vi "Shutdown.vi"(8 "error in (no error)":errorcluster, 9 "Message Data":variant, 10 "Name":string, 11 "Controller in":refnum<class "Controller.lvclass">) -> (0 "error out":errorcluster, 3 "Controller out":refnum<class "Controller.lvclass">)   [LabVIEW 2020, in "Controller.lvlib" / "Controller.lvclass"]
uses:
  Controller.lvclass
  RPC/TypeDefs/Request.ctl
  Controller.lvclass/Controller.ctl
  RPC.lvlib
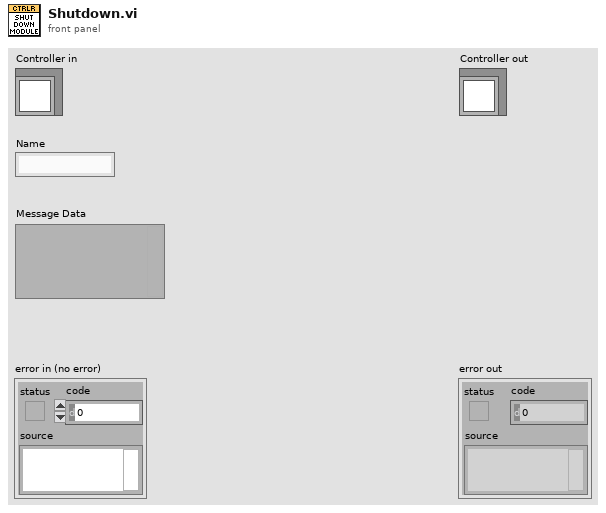
[diagram p1: front panel]
types:
  T1 = typedef "RPC.lvlib/Request.ctl" = cluster{"Method":string, "Params":variant}
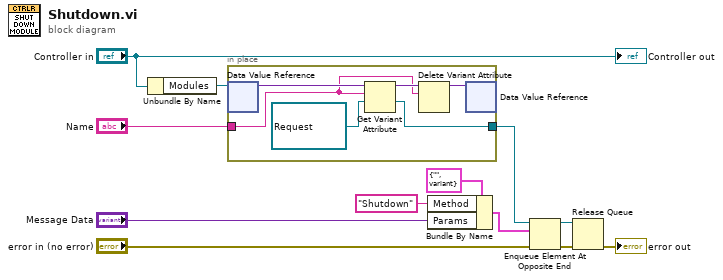
[diagram p0: block diagram]
diagram:
  n1 = Unbundle By Name("Controller in") -> ("Modules"=w10:refnum<data-value>)
  n2 = in-place {
    in-place-border: "Name" -> [w14]
    in-place-border: [w15] -> w2
    n3 = in-place-dvr #1(w10) -> (w17:variant)  [unwired: 1 out]
    n4 = Get Variant Attribute(Variant=w17, name=w14, default value (empty Variant)=refnum<queue> refnum ("queue out")) -> (duplicate Variant=w16:variant, value=w15:refnum<queue>)  [unwired: 1 in, 2 out]
    n5 = Delete Variant Attribute(6:w14, 7:w16) -> (3:w18:variant)  [unwired: 1 in, 2 out]
    n6 = in-place-dvr #1(w18) -> ()  [unwired: 2 out]
  }
  n7 = Bundle By Name(cluster=T1 {"Method"="", "Params"=variant} ("element"), "Method"="Shutdown" ("Message"), "Params"="Message Data") -> (w9:T1)
  n8 = Enqueue Element At Opposite End(queue=w2, element=w9, error in (no error)="error in (no error)") -> (queue out=w5:refnum<queue>, error out=w6:errorcluster)  [unwired: 1 in, 1 out]
  n9 = Release Queue(queue=w5, error in (no error)=w6) -> (error out=→"error out":errorcluster)  [unwired: 1 in, 2 out]
  "Controller out" <- "Controller in"
